vi "makeDecisions.vi"(8 "error in (no error)":errorcluster, 10 "model":refnum<class "Model.lvclass">, 11 "EnabledState in":refnum<class "EnabledState.lvclass">) -> (0 "error out":errorcluster, 2 "model 2":refnum<class "Model.lvclass">, 3 "EnabledState out":refnum<class "EnabledState.lvclass">)   [LabVIEW 2013, in "EnabledState.lvclass"]
uses:
  EnabledState.lvclass
  Model/Model/Model.lvclass
  Typedefs/StateSelector.ctl
  Typedefs/AITDTTypedefs.lvlib
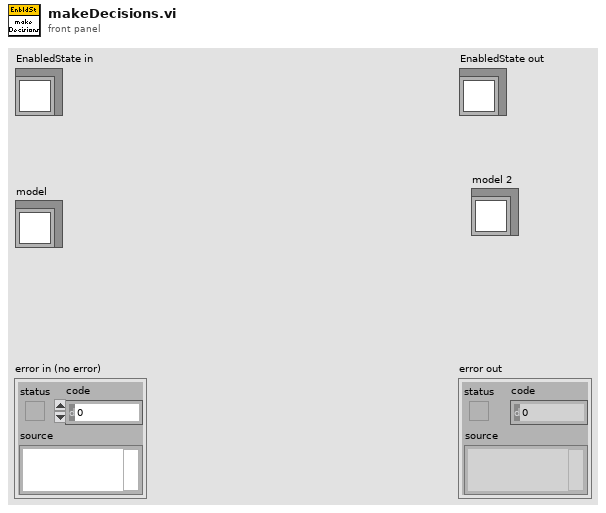
[diagram p1: front panel]
types:
  T1 = typedef "AITDTTypedefs.lvlib/StateSelector.ctl" = enum16{"AwaitingSetpointAcknowledgmentState", "EndingCycleState", "FaultState", "OffState", "PausingState", "RequestingNewSetpointState", "SamplingState", "SettlingState", "SoakingState", "StabilizingState", "StandbyState", "StoppedState", "TransitioningTemperatureState"}
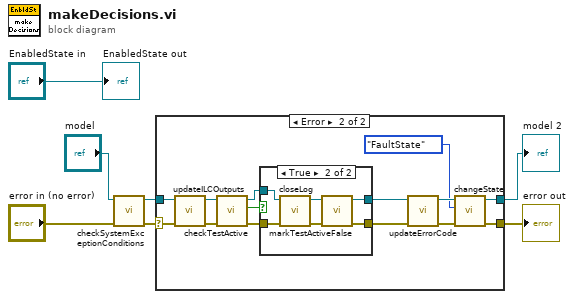
[diagram p0: block diagram]
diagram:
  n1 = call "checkSystemExceptionConditions.vi"("error in (no error)"="error in (no error)", "Model in"="model") -> ("error out"=w4:errorcluster, "Model out"=w3:refnum<class "Model.lvclass">)  [unwired: 8 in]
  n2 = case shown="Error" w4 {
    selector: w4 -> [w9 w10]
    tunnel: [w9 w21] -> w7
    tunnel: w3 -> [w8 w11]
    tunnel: [w8 w20] -> w5
    frame No Error {
    }
    frame Error {
      n3 = call "updateILCOutputs.vi"("error in (no error)"=w10, "Model in"=w11) -> ("error out"=w12:errorcluster, "Model out"=w13:refnum<class "Model.lvclass">)  [unwired: 8 in]
      n4 = call "checkTestActive.vi"("error in (no error)"=w12, "Model in"=w13) -> ("error out"=w16:errorcluster, "testActiveIsTrue"=w18:bool, "Model out"=w17:refnum<class "Model.lvclass">)  [unwired: 7 in]
      n5 = case shown="True" w18 {
        tunnel: [w25 w28] -> w14
        tunnel: [w24 w26] -> w15
        tunnel: w17 -> [w25 w31]
        tunnel: w16 -> [w24 w30]
        frame False {
        }
        frame True {
          n6 = call "closeLog.vi"("error in (no error)"=w30, "Model in"=w31) -> ("error out"=w27:errorcluster, "Model out"=w29:refnum<class "Model.lvclass">)  [unwired: 8 in]
          n7 = call "markTestActiveFalse.vi"("error in (no error)"=w27, "Model in"=w29) -> ("error out"=w26:errorcluster, "Model out"=w28:refnum<class "Model.lvclass">)  [unwired: 8 in]
        }
      }
      n8 = call "updateErrorCode.vi"("error in (no error)"=w15, "Model in"=w14) -> ("error out"=w22:errorcluster, "Model out"=w23:refnum<class "Model.lvclass">)  [unwired: 8 in]
      n9 = call "changeState.vi"("error in (no error)"=w22, "State:"=StateSelector."FaultState", "Model in"=w23) -> ("error out"=w21:errorcluster, "Model out"=w20:refnum<class "Model.lvclass">)  [unwired: 7 in]
    }
  }
  "error out" <- w7
  "model 2" <- w5
  "EnabledState out" <- "EnabledState in"
